vi "Open Document.vi"(8 "error in (no error)":errorcluster, 11 "File Path":path) -> (0 "error out":errorcluster, 3 "Document out":refnum<class "Document.lvclass">)   [LabVIEW 2017, in "LabVIEW NPOI.lvlib" / "Document.lvclass"]
doc: "Opens the <b>Document</b> file located at <b>File Path</b> for reading.\n\nNotes:\n - If <b>File Path</b> is empty (default) or is <Not A Path> or is a directory, error 7 is returned."
uses:
  Document.lvclass
  Document.lvclass/Document.ctl
  Set FilePath.vi
  Set Overwrite.vi
  <vilib>/Utility/error.llb/Error Cluster From Error Code.vi
  <vilib>/ErrorRing/Error Ring.xnode
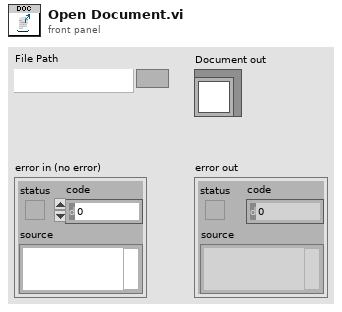
[diagram p1: front panel]
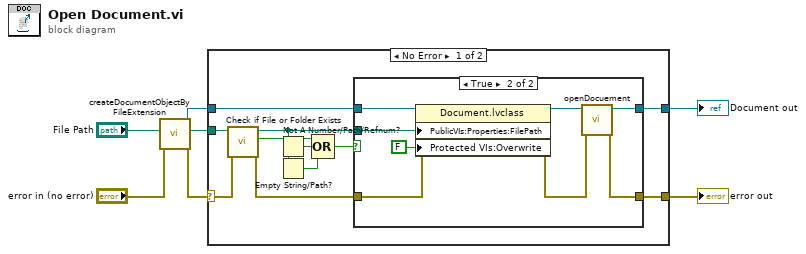
[diagram p0: block diagram]
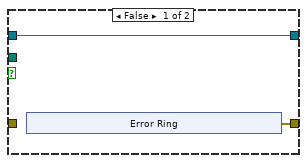
[diagram p2: hidden frame]
diagram:
  n1 = call "createDocumentObjectByFileExtension.vi"("error in (no error)"="error in (no error)", "File Path"="File Path") -> ("error out"=w1:errorcluster, "File Path dup"=w3:path, "Document out"=w4:refnum<class "Document.lvclass">)  [unwired: 7 in]
  n2 = case shown="No Error" w1 {
    selector: w1 -> [w14 w34]
    tunnel: [w16 w34] -> w7
    tunnel: [w17 w33] -> w6
    tunnel: w4 -> [w18 w33]
    tunnel: w3 -> [w15 _]
    frame No Error {
      n3 = call <vilib>:"Check if File or Folder Exists.vi"("error in (no error)"=w14, "path"=w15) -> ("error out"=w13:errorcluster, "file or folder exists?"=w9:bool, "dup path"=w10:path)  [unwired: 7 in]
      n4 = Not A Number/Path/Refnum?(number/path/refnum=w10) -> (NaN/Path/Refnum?=w12:bool)
      n5 = Empty String/Path?(string/path=w10) -> (empty?=w11:bool)
      n6 = Compound Arithmetic op=OR(w9, w12, w11) -> (w8:bool)
      n7 = case shown="True" w8 {
        tunnel: w18 -> [w20 w30]
        tunnel: [w20 w32] -> w17
        tunnel: [w19 w31] -> w16
        tunnel: w13 -> [_ w27]
        tunnel: w10 -> [_ w28]
        frame False {
          n8 = xnode "Error Ring"() -> ("error out"=w19:errorcluster)
        }
        frame True {
          n9 = property class="Document.lvclass"(reference=w30, error in=w27, "PublicVIs:Properties:FilePath"=w28, "Protected VIs:Overwrite"=FALSE ("Overwrite")) -> (reference out=w29:refnum<class "Document.lvclass">, error out=w26:errorcluster)
          n10 = call-dynamic "openDocuement.vi"("error in (no error)"=w26, "Document in"=w29) -> ("error out"=w31:errorcluster, "Document out"=w32:refnum<class "Document.lvclass">)  [unwired: 8 in]
        }
      }
    }
    frame Error {
    }
  }
  "error out" <- w7
  "Document out" <- w6
